vi "_TangoAttributeDataReadyEventGroupCreate.vi"(0 "error in":errorcluster) -> (1 "attribute data ready event ref":T1, 2 "error out":errorcluster)   [LabVIEW 2014, in "tango.lvlib"]
uses:
  tango.lvlib
  Common VIs/Typedefs/_AttributeDataReadyEventRef.ctl
  tango_binding.so
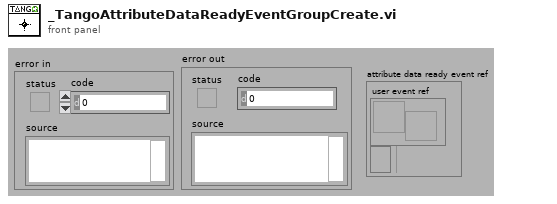
[diagram p1: front panel]
types:
  T1 = typedef "tango.lvlib/_AttributeDataReadyEventRef.ctl" = cluster{"user event ref":refnum<user-event>, "user event reg refnum":refnum<event-registration>}
  T2 = typedef "tango.lvlib/_AttributeDataReady_t.ctl" = cluster{"device name":string, "attribute name":string, "attribute data type":i16, "data counter":i16}
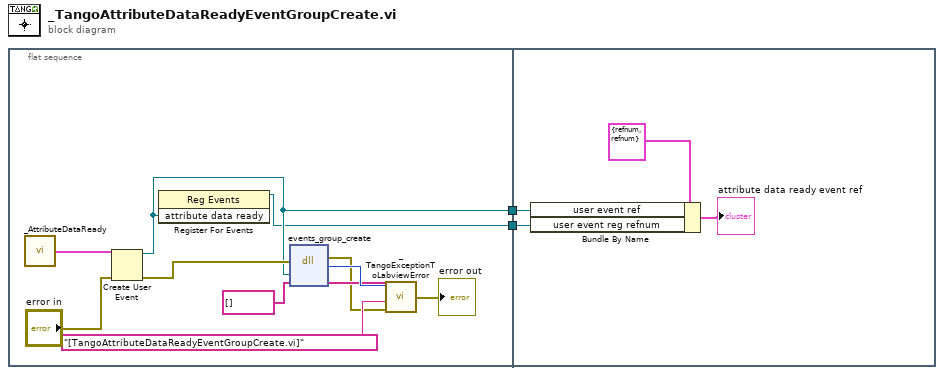
[diagram p0: block diagram]
diagram:
  n1 = flat-sequence {
    tunnel: [w5] -> w2
    tunnel: [w4] -> w1
    tunnel: w2 -> [w16]
    tunnel: w1 -> [w15]
    frame #0 {
      n2 = call "_AttributeDataReady.vi"() -> ("attribute data ready"=w3:T2)
      n3 = Create User Event(user event datatype=w3, error in="error in") -> (user event=w5:refnum<user-event>, error out=w12:errorcluster)
      n4 = register-events(w5) -> (reference out=w4:refnum<event-registration>)  [unwired: 2 in, 1 out]
      n5 = dll-call lib="tango_binding.*" fn="events_group_create"(error in=w12, "event refnum"=w5, "error_stack"=string[] []) -> (error out=w6:errorcluster, "return type"=w10:i32, "error_stack"=w9:string[])  [unwired: 3 in, 1 out]
      n6 = call "_TangoExceptionToLabviewError.vi"("error in"=w6, "location"="[TangoAttributeDataReadyEventGroupCreate.vi]", "error stack"=w9, "error code"=w10) -> ("error out"=→"error out":errorcluster)
    }
    frame #1 {
      n7 = Bundle By Name(cluster=T1 {"user event ref"=refnum, "user event reg refnum"=refnum} ("input cluster"), "user event ref"=w16, "user event reg refnum"=w15) -> (→"attribute data ready event ref":T1)
    }
  }
